vi "Calibration Scaling (Read).vi"(6 "ISOBUS address":T3=-1 caption="ISOBUS address (-1)", 8 "error in":errorcluster, 11 "Mercury Reference In":T4) -> (0 "error out":errorcluster, 1 "Unit":T1, 2 "Scaling Factor":dbl, 3 "Mercury Reference Out":T4, 4 "Valid?":T2)   [LabVIEW 2013, in "Mercury iXX.lvlib" / "Pressure.lvlib"]
doc: "Read the current value of the pressure scaling factor."
uses:
  <instrlib>/Mercury iXX/Public/Libraries/Pressure.lvlib
  <instrlib>/Mercury iXX/Public/Controls/Mercury Reference.ctl
  <instrlib>/Mercury iXX/Public/Controls/Comms Transport Layer.ctl
  <instrlib>/Mercury iXX/Private/Controls/Query Dynamic Reference.ctl
  <instrlib>/Mercury iXX/Public/Controls/ISOBus Address.ctl
  <instrlib>/Mercury iXX/Public/Controls/Is Valid LED.ctl
  <instrlib>/Mercury iXX/Public/Controls/Unit String.ctl
  <instrlib>/Mercury iXX/Private/Controls/Command Verbs.ctl
  <instrlib>/Mercury iXX/Mercury iXX.lvlib
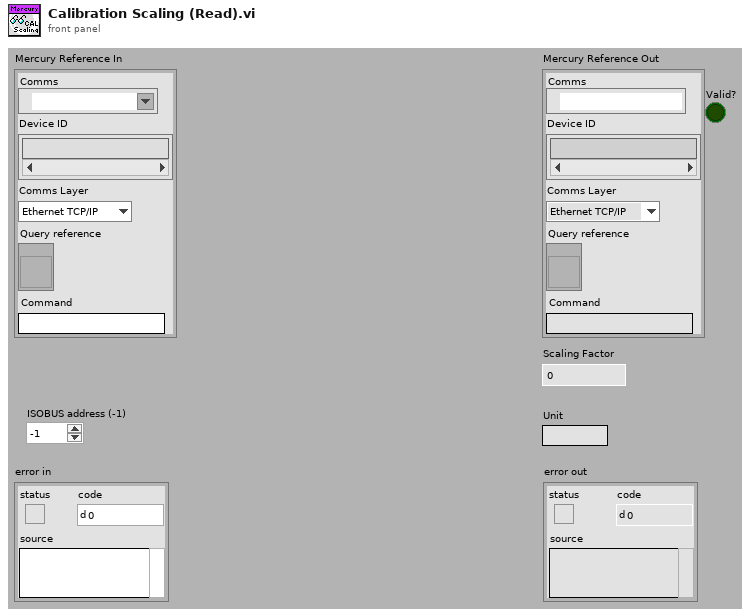
[diagram p1: front panel]
types:
  T1 = typedef "Mercury iXX.lvlib/Unit String.ctl" = string
  T2 = typedef "Mercury iXX.lvlib/Is Valid LED.ctl" = bool
  T3 = typedef "Mercury iXX.lvlib/ISOBus Address.ctl" = i32
  T4 = typedef "Mercury iXX.lvlib/Mercury Reference.ctl" = cluster{"Comms":refnum<visa-resource-name>, "Device ID":string[], "Comms Layer":T5, "Command":string, "Query reference":T6}
  T5 = typedef "Mercury iXX.lvlib/Comms Transport Layer.ctl" = enum16{"Ethernet TCP/IP", "USB", "ISOBus - RS-232", "GPIB"}
  T6 = typedef "Mercury iXX.lvlib/Query Dynamic Reference.ctl" = refnum<vi>
  T7 = typedef "Mercury iXX.lvlib/Command Verbs.ctl" = string
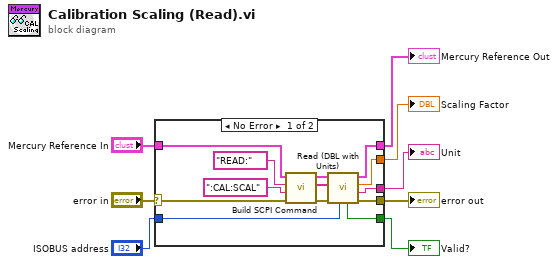
[diagram p0: block diagram]
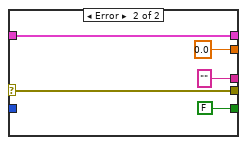
[diagram p2: hidden frame]
diagram:
  n1 = case shown="No Error" "error in" {
    selector: "error in" -> [w11 w26]
    tunnel: "Mercury Reference In" -> [w18 w25]
    tunnel: [w17 w25] -> w7
    tunnel: [w16 w26] -> w6
    tunnel: [w15 T1 "" ("Unit")] -> w5
    tunnel: [w14 0.0 ("Data (Dbl)")] -> w4
    tunnel: "ISOBUS address" -> [w10 _]
    tunnel: [w9 T2 FALSE ("Valid?")] -> w1
    frame No Error {
      n2 = call <instrlib>:"Build SCPI Command.vi"("error in"=w11, "Noun(s)"=":CAL:SCAL" ("Command"), "Verb"=T7 "READ:", "Mercury Reference In"=w18) -> ("error out"=w13:errorcluster, "SCPI Message(s)"=w20:string[], "Mercury Reference Out"=w21:T4)  [unwired: 5 out]
      n3 = call <instrlib>:"Read (DBL with Units).vi"("ISOBUS address"=w10, "error in"=w13, "SCPI Message(s)"=w20, "Mercury Reference In"=w21) -> ("error out"=w16:errorcluster, "Unit"=w15:T1, "Data (Dbl)"=w14:dbl, "Mercury Reference Out"=w17:T4, "Valid?"=w9:T2)  [unwired: 3 out]
    }
    frame Error {
    }
  }
  "Mercury Reference Out" <- w7
  "error out" <- w6
  "Scaling Factor" <- w4
  "Valid?" <- w1
  "Unit" <- w5
